vi "Color_Levelmeter.vi"(1 "In":i32) -> (0 "Out":i32)   [LabVIEW 2016]
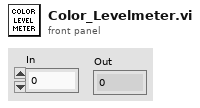
[diagram p1: front panel]
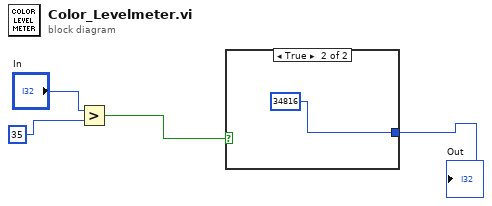
[diagram p0: block diagram]
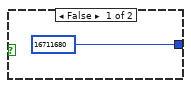
[diagram p2: hidden frame]
diagram:
  n1 = Greater?(x="In", y=35) -> (0:w2:bool)
  n2 = case shown="True" w2 {
    tunnel: [16711680 34816] -> w1
    frame False {
    }
    frame True {
    }
  }
  "Out" <- w1
